vi "WriteCustomData.vi"(8 "error in":errorcluster, 9 "Data":string, 10 "Key":string, 11 "Image Reference In":T1) -> (0 "error out":errorcluster, 3 "Image Reference Out":T1)   [LabVIEW 2024, in "OpenLvVision_Image.lvlib" / "Management.lvlib"]
doc: "Write the provided data with the specified key in the image's data. \nIf the key is new, it's added; otherwise, its existing value is updated."
uses:
  Management.lvlib
  TypeDef/Image.ctl
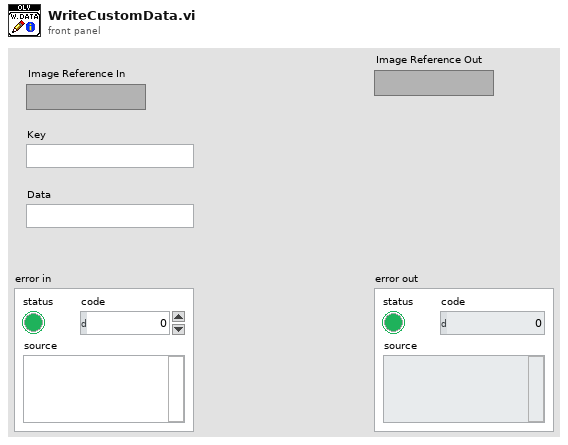
[diagram p1: front panel]
types:
  T1 = typedef "OpenLvVision_Image.lvlib/Management.lvlib/Image.ctl" = refnum<image>
  T2 = typedef "IMAQ Image.ctl" = refnum<image>
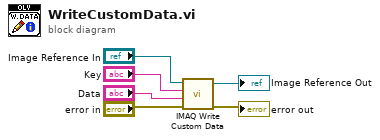
[diagram p0: block diagram]
diagram:
  n1 = call "IMAQ Write Custom Data"("error in (no error)"="error in", "Custom Data In"="Data", "Key"="Key", "Image"="Image Reference In") -> ("error out"=→"error out":errorcluster, "Image Out"=→"Image Reference Out":T2)  [unwired: 6 in]
